vi "Write TOML File (TOML).vi"(8 "error in (no error)":errorcluster, 10 "Value":T1, 11 "file path (use dialog)":path) -> (0 "error out":errorcluster)   [LabVIEW 2017, in "TOML.lvlib"]
uses:
  TOML.lvlib
  TOML Value.ctl
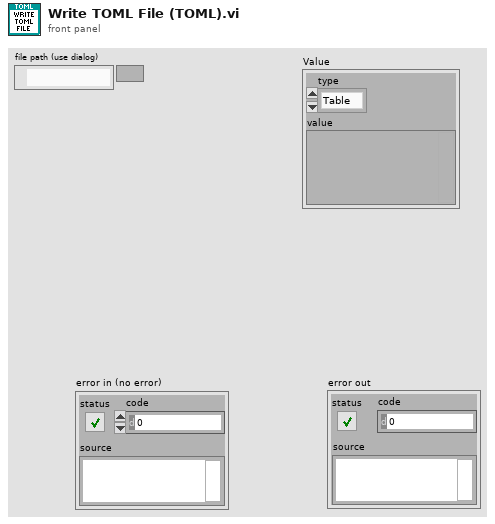
[diagram p1: front panel]
types:
  T1 = typedef "TOML.lvlib/TOML Value.ctl" = cluster{"type":enum16{"Table", "Array", "String", "Integer", "Float", "Boolean", "Offset Date-Time", "Local Date-Time", "Local Date", "Local Time"}, "value":variant}
  T2 = enum16{"open", "replace", "create", "open or create", "replace or create", "replace or create with confirmation"}
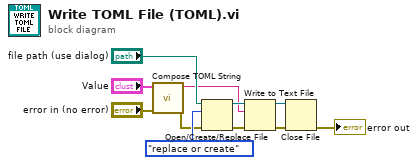
[diagram p0: block diagram]
diagram:
  n1 = call "Compose TOML String.vi"("error in (no error)"="error in (no error)", "Value"="Value") -> ("error out"=w2:errorcluster, "String"=w1:string)  [unwired: 8 in]
  n2 = Open/Create/Replace File(file path (use dialog)="file path (use dialog)", error in=w2, operation (0:open)=T2."replace or create") -> (refnum out=w8:refnum<file>, error out=w9:errorcluster)  [unwired: 3 in, 1 out]
  n3 = Write to Text File(file (use dialog)=w8, text=w1, error in=w9) -> (refnum out=w6:refnum<file>, error out=w7:errorcluster)  [unwired: 1 in, 1 out]
  n4 = Close File(refnum=w6, error in=w7) -> (error out=→"error out":errorcluster)  [unwired: 1 out]
